vi "Write Port Ref.vi"(8 "error in (no error)":errorcluster, 10 "Port Ref":refnum<visa-resource-name>, 11 "RS232 in":refnum<class "RS-xxx.lvclass">) -> (0 "error out":errorcluster, 3 "RS232 out":refnum<class "RS-xxx.lvclass">)   [LabVIEW 2023, in "Protocols.lvlib" / "RS-xxx.lvclass"]
uses:
  RS-xxx.lvclass
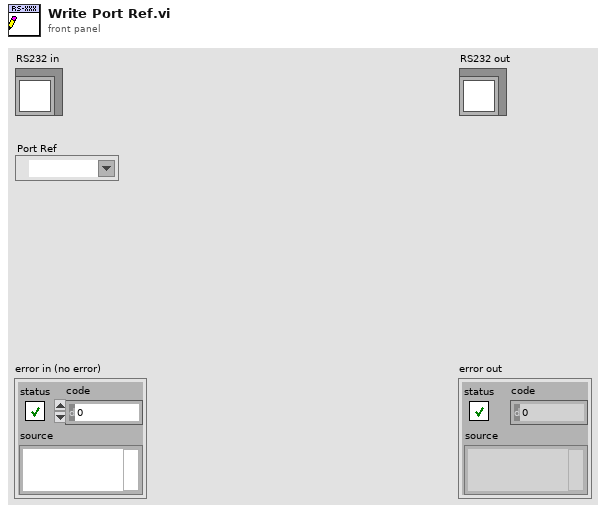
[diagram p1: front panel]
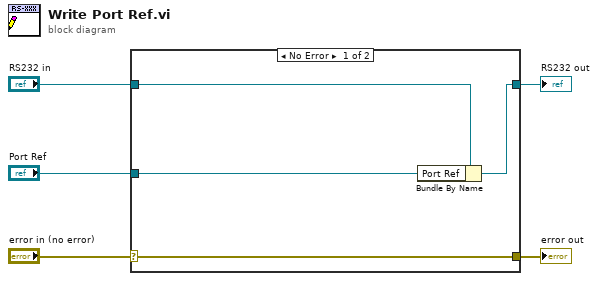
[diagram p0: block diagram]
diagram:
  n1 = case shown="No Error" "error in (no error)" {
    selector: "error in (no error)" -> [w9 w10]
    tunnel: [w9 w10] -> w4
    tunnel: [w7 w11] -> w2
    tunnel: "RS232 in" -> [w8 w11]
    tunnel: "Port Ref" -> [w6 _]
    frame No Error {
      n2 = Bundle By Name(cluster=w8, "Port Ref"=w6) -> (w7:refnum<class "RS-xxx.lvclass">)
    }
    frame Error {
    }
  }
  "error out" <- w4
  "RS232 out" <- w2
